vi "Plot Pole-Zero.vi"   [LabVIEW 2016]
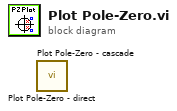
[diagram p0: block diagram]
diagram:
  n1 = call "Plot Pole-Zero - cascade.vi"() -> ()  [unwired: 5 in, 1 out]
  n2 = call "Plot Pole-Zero - direct.vi"() -> ()  [unwired: 5 in, 1 out]
